vi "FT10_Fornax Read Power.vi"(10 "Auto Set Power Cluster in":T2, 11 "Message Handling Cluster in":T6={"Fornax Connected?"=refnum, "Unitherm Connected?"=refnum, "M4X Connected?"=refnum, "Unitherm Connect/Disconnect"=refnum, "Fornax Connection"=refnum, "UNITHERM Connection"="", "M4X Connection"=0, "FPGA VI Reference Out"=refnum, "PXI-7854R Connected?"=refnum, "Fornax Connect/Disconnect"=refnum, "7854 Connect/Disconnect"=refnum, "M4X Connect/Disconnect"=refnum, "Config cluster"={"Unitherm Port"="COM4", "Simulate Values"=TRUE, "Fornax Connect Attempts"=0}, "Log Queue"=refnum, "Log Analysis Cluster - Current"={"RMS"=0.0, "Envelope Frequency"=0.0, "Peak"=0.0, "Crest Factor"=0.0, "Duty Cyle %"=0.0, "P-P"=0.0, "Frequency"=0.0, "THD"=0.0, "Postive Peak"=0.0, "Negative Peak"=0.0, "Mag_H1"=0.0, "Phase_H1"=0.0, "Mag_H3"=0.0, "Phase_H3"=0.0, "Mag_H5"=0.0, "Phase_H5"=0.0}, "Log Waveform Cluster - Current"={"t0"=timestamp(0 s since 1904-01-01), "dt"=1.0, "Y"=[]}, "Log Time"=timestamp(0 s since 1904-01-01), "Log Flag"=FALSE, "Log - Activation Settings Cluster"={"Log - Unitherm Load"="", "Log - Port"="", "Log - Mode"="", "Log - Power Level"=""}, "Log - Port Mode Cluster"={"Mono1 Cut Enum"=enum."Pure", "Mono2 Cut Enum"=enum."Pure", "Mono1 Coag Enum"=enum."Spray", "Mono2 Coag Enum"=enum."Spray", "Bipolar Enum"=enum."Standard"}, "Log Analysis Cluster - Diff Voltage"={"RMS"=0.0, "Envelope Frequency"=0.0, "Peak"=0.0, "Crest Factor"=0.0, "Duty Cyle %"=0.0, "P-P"=0.0, "Frequency"=0.0, "THD"=0.0, "Postive Peak"=0.0, "Negative Peak"=0.0, "Mag_H1"=0.0, "Phase_H1"=0.0, "Mag_H3"=0.0, "Phase_H3"=0.0, "Mag_H5"=0.0, "Phase_H5"=0.0}, "Log Waveform Cluster - Diff Voltage"={"t0"=timestamp(0 s since 1904-01-01), "dt"=1.0, "Y"=[]}, "Indicator Cluster"={"Mono1 - Cut Power"=refnum, "Mono1 - Coag Power"=refnum, "Mono2 - Cut Power"=refnum, "Mono2 - Coag Power"=refnum, "Bipolar Power"=refnum, "Mono1 Cut Enum"=refnum, "Mono1 Coag Enum"=refnum, "Mono2 Cut Enum"=refnum, "Mono2 Coag Enum"=refnum, "Bipolar Enum"=refnum}, "Log Power Level Cluster"={"Log Mono1 Cut Power"="", "Log Mono1 Coag Power"="", "Log Mono2 Cut Power"="", "Log Mono2 Coag Power"="", "Log Bipolar Power"=""}, "Footswitch Cluster"={"PXI-2565 reset device (boolean value)"=TRUE, "topology name"="2565/16-SPST", "PXI-2565 simulate (boolean value)"=FALSE, "PXI-2565 resource name"=""}}) -> (2 "Auto Set Power Cluster out":T2, 3 "Message Handling Cluster out":T6={"Fornax Connected?"=refnum, "Unitherm Connected?"=refnum, "M4X Connected?"=refnum, "Unitherm Connect/Disconnect"=refnum, "Fornax Connection"=refnum, "UNITHERM Connection"="", "M4X Connection"=0, "FPGA VI Reference Out"=refnum, "PXI-7854R Connected?"=refnum, "Fornax Connect/Disconnect"=refnum, "7854 Connect/Disconnect"=refnum, "M4X Connect/Disconnect"=refnum, "Config cluster"={"Unitherm Port"="COM4", "Simulate Values"=TRUE, "Fornax Connect Attempts"=0}, "Log Queue"=refnum, "Log Analysis Cluster - Current"={"RMS"=0.0, "Envelope Frequency"=0.0, "Peak"=0.0, "Crest Factor"=0.0, "Duty Cyle %"=0.0, "P-P"=0.0, "Frequency"=0.0, "THD"=0.0, "Postive Peak"=0.0, "Negative Peak"=0.0, "Mag_H1"=0.0, "Phase_H1"=0.0, "Mag_H3"=0.0, "Phase_H3"=0.0, "Mag_H5"=0.0, "Phase_H5"=0.0}, "Log Waveform Cluster - Current"={"t0"=timestamp(0 s since 1904-01-01), "dt"=1.0, "Y"=[]}, "Log Time"=timestamp(0 s since 1904-01-01), "Log Flag"=FALSE, "Log - Activation Settings Cluster"={"Log - Unitherm Load"="", "Log - Port"="", "Log - Mode"="", "Log - Power Level"=""}, "Log - Port Mode Cluster"={"Mono1 Cut Enum"=enum."Pure", "Mono2 Cut Enum"=enum."Pure", "Mono1 Coag Enum"=enum."Spray", "Mono2 Coag Enum"=enum."Spray", "Bipolar Enum"=enum."Standard"}, "Log Analysis Cluster - Diff Voltage"={"RMS"=0.0, "Envelope Frequency"=0.0, "Peak"=0.0, "Crest Factor"=0.0, "Duty Cyle %"=0.0, "P-P"=0.0, "Frequency"=0.0, "THD"=0.0, "Postive Peak"=0.0, "Negative Peak"=0.0, "Mag_H1"=0.0, "Phase_H1"=0.0, "Mag_H3"=0.0, "Phase_H3"=0.0, "Mag_H5"=0.0, "Phase_H5"=0.0}, "Log Waveform Cluster - Diff Voltage"={"t0"=timestamp(0 s since 1904-01-01), "dt"=1.0, "Y"=[]}, "Indicator Cluster"={"Mono1 - Cut Power"=refnum, "Mono1 - Coag Power"=refnum, "Mono2 - Cut Power"=refnum, "Mono2 - Coag Power"=refnum, "Bipolar Power"=refnum, "Mono1 Cut Enum"=refnum, "Mono1 Coag Enum"=refnum, "Mono2 Cut Enum"=refnum, "Mono2 Coag Enum"=refnum, "Bipolar Enum"=refnum}, "Log Power Level Cluster"={"Log Mono1 Cut Power"="", "Log Mono1 Coag Power"="", "Log Mono2 Cut Power"="", "Log Mono2 Coag Power"="", "Log Bipolar Power"=""}, "Footswitch Cluster"={"PXI-2565 reset device (boolean value)"=TRUE, "topology name"="2565/16-SPST", "PXI-2565 simulate (boolean value)"=FALSE, "PXI-2565 resource name"=""}}, 5 "For Loop Iterations":T1)   [LabVIEW 2024]
uses:
  Controls/Control_Message Handling Cluster.ctl
  Controls/Control_M4X Connection.ctl
  Controls/Control_PXI-7854R FPGA Reference.ctl
  Controls/Control_Config Cluster.ctl
  Controls/Control_Config Unitherm Port.ctl
  Controls/Control_Config Simulate Values.ctl
  Controls/Control_Config Fornax Connect Attempts.ctl
  Controls/Control_Log Queue.ctl
  Controls/Control_Log Cluster.ctl
  Controls/Control_Log Time.ctl
  Controls/Control_Log Waveform Cluster - Current.ctl
  Controls/Control_Log Analysis Cluster - Current.ctl
  Controls/Control_Log Activation Settings Cluster.ctl
  Controls/Control_Log Unitherm Load.ctl
  Controls/Control_Log Port.ctl
  Controls/Control_Log Mode.ctl
  Controls/Control_Log Power Level.ctl
  Controls/Control_Log Waveform Cluster - Diff Voltage.ctl
  Controls/Control_Log Analysis Cluster - Diff Voltage.ctl
  Controls/Control_Log Flag.ctl
  Controls/Control_Log Port Mode Cluster.ctl
  Controls/Control_Fornax Mono1 Cut Enum.ctl
  Controls/Control_Fornax Mono2 Cut Enum.ctl
  Controls/Control_Fornax Mono1 Coag Enum.ctl
  Controls/Control_Fornax Mono2 Coag Enum.ctl
  Controls/Control_Fornax Bipolar Enum.ctl
  Controls/Control_Indicator Cluster.ctl
  Controls/Control_Log Power Level Cluster.ctl
  Controls/Control_Log Mono1 Cut Power.ctl
  Controls/Control_Log Mono1 Coag Power.ctl
  Controls/Control_Log Mono2 Cut Power.ctl
  Controls/Control_Log Mono2 Coag Power.ctl
  Controls/Control_Log Bipolar Power.ctl
  Controls/Control_Footswitch Reset Device Bool.ctl
  <instrlib>/niSwitch/niSwitch.llb/niSwitch Topologies.ctl
  Controls/Control_Footswitch Simulate Bool.ctl
  Controls/Control_Footswitch Resource Name.ctl
  Controls/Control_Auto Set Power Cluster.ctl
  Controls/Control_Semi-Auto Port.ctl
  Controls/Control_Semi-Auto Mode.ctl
  Controls/Control_Semi-Auto Power Level.ctl
  Controls/Control_Semi-Auto Power Level - For Loop Iterations.ctl
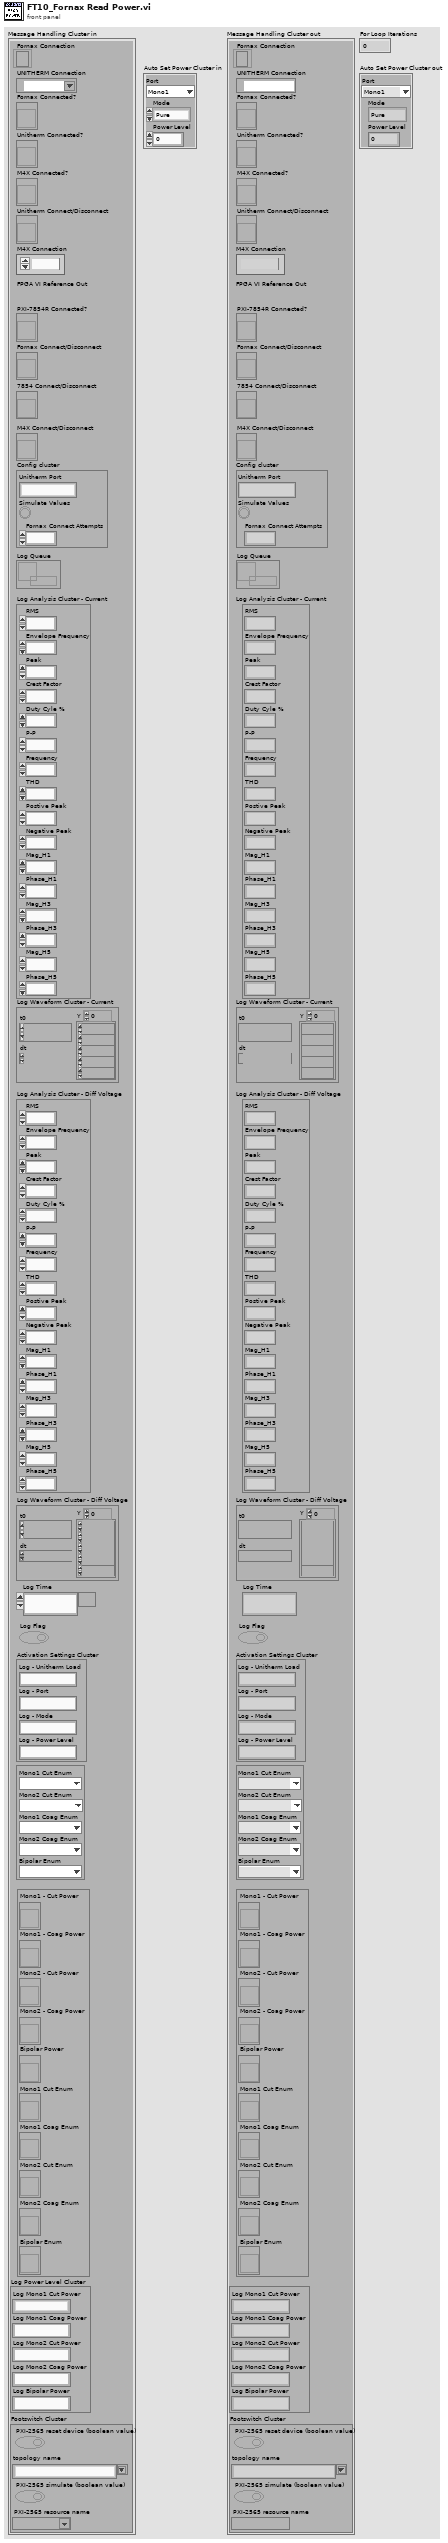
[diagram p1: front panel]
types:
  T1 = typedef "Control_Semi-Auto Power Level - For Loop Iterations.ctl" = i32
  T2 = typedef "Control_Auto Set Power Cluster.ctl" = cluster{"Port":T3, "Mode":T4, "Power Level":T5}
  T3 = typedef "Control_Semi-Auto Port.ctl" = enum16{"Mono1", "Mono2", "Bipolar", "Ligasure", "Error"}
  T4 = typedef "Control_Semi-Auto Mode.ctl" = enum16{"Pure", "Blend", "Spray", "Fulgerate", "Standard", "Macro", "Precision", "Ligasure", "Error"}
  T5 = typedef "Control_Semi-Auto Power Level.ctl" = dbl
  T6 = typedef "Control_Message Handling Cluster.ctl" = cluster{"Fornax Connected?":refnum<vi>, "Unitherm Connected?":refnum<vi>, "M4X Connected?":refnum<vi>, "Unitherm Connect/Disconnect":refnum<vi>, "Fornax Connection":refnum<k5>, "UNITHERM Connection":refnum<visa-resource-name>, "M4X Connection":T7, "FPGA VI Reference Out":T8, "PXI-7854R Connected?":refnum<vi>, "Fornax Connect/Disconnect":refnum<vi>, "7854 Connect/Disconnect":refnum<vi>, "M4X Connect/Disconnect":refnum<vi>, "Config cluster":T9, "Log Queue":T13, "Log Analysis Cluster - Current":T14, "Log Waveform Cluster - Current":T15, "Log Time":T16, "Log Flag":T17, "Log - Activation Settings Cluster":T18, "Log - Port Mode Cluster":T23, "Log Analysis Cluster - Diff Voltage":T29, "Log Waveform Cluster - Diff Voltage":T30, "Indicator Cluster":T31, "Log Power Level Cluster":T32, "Footswitch Cluster":cluster{"PXI-2565 reset device (boolean value)":T38, "topology name":T39, "PXI-2565 simulate (boolean value)":T40, "PXI-2565 resource name":T41}}
  T7 = typedef "Control_M4X Connection.ctl" = u32
  T8 = typedef "Control_PXI-7854R FPGA Reference.ctl" = refnum<k20>
  T9 = typedef "Control_Config Cluster.ctl" = cluster{"Unitherm Port":T10, "Simulate Values":T11, "Fornax Connect Attempts":T12}
  T10 = typedef "Control_Config Unitherm Port.ctl" = string
  T11 = typedef "Control_Config Simulate Values.ctl" = bool
  T12 = typedef "Control_Config Fornax Connect Attempts.ctl" = i32
  T13 = typedef "Control_Log Queue.ctl" = refnum<queue>
  T14 = typedef "Control_Log Analysis Cluster - Current.ctl" = cluster{"RMS":dbl, "Envelope Frequency":dbl, "Peak":dbl, "Crest Factor":dbl, "Duty Cyle %":dbl, "P-P":dbl, "Frequency":dbl, "THD":dbl, "Postive Peak":dbl, "Negative Peak":dbl, "Mag_H1":dbl, "Phase_H1":dbl, "Mag_H3":dbl, "Phase_H3":dbl, "Mag_H5":dbl, "Phase_H5":dbl}
  T15 = typedef "Control_Log Waveform Cluster - Current.ctl" = waveform(dbl)
  T16 = typedef "Control_Log Time.ctl" = timestamp
  T17 = typedef "Control_Log Flag.ctl" = bool
  T18 = typedef "Control_Log Activation Settings Cluster.ctl" = cluster{"Log - Unitherm Load":T19, "Log - Port":T20, "Log - Mode":T21, "Log - Power Level":T22}
  T19 = typedef "Control_Log Unitherm Load.ctl" = string
  T20 = typedef "Control_Log Port.ctl" = string
  T21 = typedef "Control_Log Mode.ctl" = string
  T22 = typedef "Control_Log Power Level.ctl" = string
  T23 = typedef "Control_Log Port Mode Cluster.ctl" = cluster{"Mono1 Cut Enum":T24, "Mono2 Cut Enum":T25, "Mono1 Coag Enum":T26, "Mono2 Coag Enum":T27, "Bipolar Enum":T28}
  T24 = typedef "Control_Fornax Mono1 Cut Enum.ctl" = enum16{"Pure", "Blend"}
  T25 = typedef "Control_Fornax Mono2 Cut Enum.ctl" = enum16{"Pure", "Blend"}
  T26 = typedef "Control_Fornax Mono1 Coag Enum.ctl" = enum16{"Fulgerate", "Spray"}
  T27 = typedef "Control_Fornax Mono2 Coag Enum.ctl" = enum16{"Fulgerate", "Spray"}
  T28 = typedef "Control_Fornax Bipolar Enum.ctl" = enum16{"Standard", "Macro", "Precision"}
  T29 = typedef "Control_Log Analysis Cluster - Diff Voltage.ctl" = cluster{"RMS":dbl, "Envelope Frequency":dbl, "Peak":dbl, "Crest Factor":dbl, "Duty Cyle %":dbl, "P-P":dbl, "Frequency":dbl, "THD":dbl, "Postive Peak":dbl, "Negative Peak":dbl, "Mag_H1":dbl, "Phase_H1":dbl, "Mag_H3":dbl, "Phase_H3":dbl, "Mag_H5":dbl, "Phase_H5":dbl}
  T30 = typedef "Control_Log Waveform Cluster - Diff Voltage.ctl" = waveform(dbl)
  T31 = typedef "Control_Indicator Cluster.ctl" = cluster{"Mono1 - Cut Power":refnum<vi>, "Mono1 - Coag Power":refnum<vi>, "Mono2 - Cut Power":refnum<vi>, "Mono2 - Coag Power":refnum<vi>, "Bipolar Power":refnum<vi>, "Mono1 Cut Enum":refnum<vi>, "Mono1 Coag Enum":refnum<vi>, "Mono2 Cut Enum":refnum<vi>, "Mono2 Coag Enum":refnum<vi>, "Bipolar Enum":refnum<vi>}
  T32 = typedef "Control_Log Power Level Cluster.ctl" = cluster{"Log Mono1 Cut Power":T33, "Log Mono1 Coag Power":T34, "Log Mono2 Cut Power":T35, "Log Mono2 Coag Power":T36, "Log Bipolar Power":T37}
  T33 = typedef "Control_Log Mono1 Cut Power.ctl" = string
  T34 = typedef "Control_Log Mono1 Coag Power.ctl" = string
  T35 = typedef "Control_Log Mono2 Cut Power.ctl" = string
  T36 = typedef "Control_Log Mono2 Coag Power.ctl" = string
  T37 = typedef "Control_Log Bipolar Power.ctl" = string
  T38 = typedef "Control_Footswitch Reset Device Bool.ctl" = bool
  T39 = typedef "niSwitch Topologies.ctl" = string
  T40 = typedef "Control_Footswitch Simulate Bool.ctl" = bool
  T41 = typedef "Control_Footswitch Resource Name.ctl" = refnum<k15>
  T42 = typedef "Control_Semi-Auto Power Level - Change Power Cluster.ctl" = cluster{"Valid?":T43, "For Loop Iterations":T1}
  T43 = typedef "Control_Semi-Auto Power Level - Valid" = bool
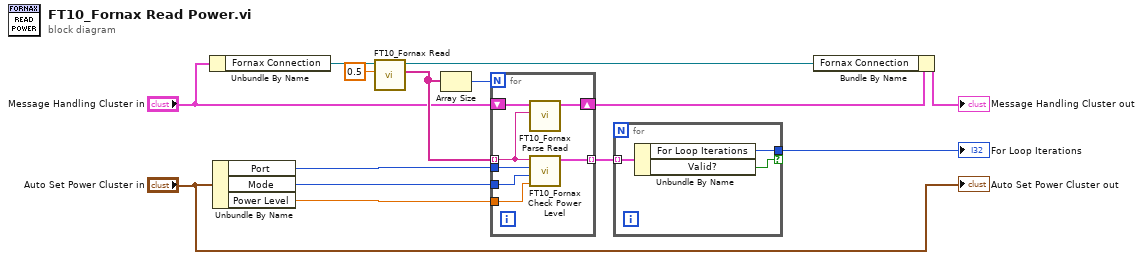
[diagram p0: block diagram]
diagram:
  n1 = Unbundle By Name("Message Handling Cluster in") -> ("Fornax Connection"=w12:refnum<k5>)
  n2 = Unbundle By Name("Auto Set Power Cluster in") -> ("Port"=w7:T3, "Mode"=w6:T4, "Power Level"=w5:T5)
  n3 = call "FT10_Fornax Read.vi"("Timeout"=0.5, "TCP Network Connection in"=w12) -> ("JSON Message"=w11:string[], "TCP Network Connection out"=w14:refnum<k5>)  [unwired: 7 in, 1 out]
  n4 = Array Size(array=w11) -> (size(s)=w10:i32)
  n5 = for {
    N: w10 -> [_]
    tunnel: w11 -> [w15] mode=indexing
    tunnel: w7 -> [w21]
    tunnel: w6 -> [w20]
    tunnel: w5 -> [w19]
    tunnel: [w18] -> w4 mode=indexing
    shift-right: [w16] -> w1
    shift-left: "Message Handling Cluster in" -> [w17]
    n6 = call "FT10_Fornax Parse Read.vi"("JSON in"=w15, "Message Handling Cluster in"=w17) -> ("Message Handling Cluster out"=w16:T6)  [unwired: 8 in, 1 out]
    n7 = call "FT10_Fornax Check Power Level.vi"("Power Level in"=w19, "Mode in"=w20, "Port in"=w21, "JSON in"=w15) -> ("output cluster"=w18:T42)  [unwired: 7 in]
  }
  n8 = for {
    tunnel: w4 -> [w24] mode=indexing
    tunnel: [w23] -> w3 if=w22
    n9 = Unbundle By Name(w24) -> ("For Loop Iterations"=w23:T1, "Valid?"=w22:T43)
  }
  "For Loop Iterations" <- w3
  n10 = Bundle By Name(cluster=w1, "Fornax Connection"=w14) -> (→"Message Handling Cluster out":T6)
  "Auto Set Power Cluster out" <- "Auto Set Power Cluster in"
